vi "MergeOverrideViWithMethod.vi"(0 "ViRef":refnum<vi>, 1 "OverrideVIRef":refnum<vi>, 2 "GetControlNamesThatShouldBeIgnored":string[](array[string]), 5 "error in":errorcluster) -> (19 "error out":errorcluster)   [LabVIEW 2020, in "ClassWriterNative.lvclass"]
uses:
  <resource>/Framework/Providers/Open_GDS/ClassProviders/Provider_LvNativeClass/ClassWriterNative_class/ClassWriterNative.lvclass
  <vilib>/Utility/miscctls.llb/LVPositionTypeDef.ctl
  <resource>/Framework/Providers/Open_GDS/ClassProviders/Provider_LvNativeClass/ClassWriterNative_class/ClassWriterNative.lvclass/ClassWriterNative.ctl
  <userlib>/_OpenG.lib/error/error.llb/openg_error.lvlib
panel:
  out "These CP Termibnlas should not be connected to an controls":i32[](array[numeric])
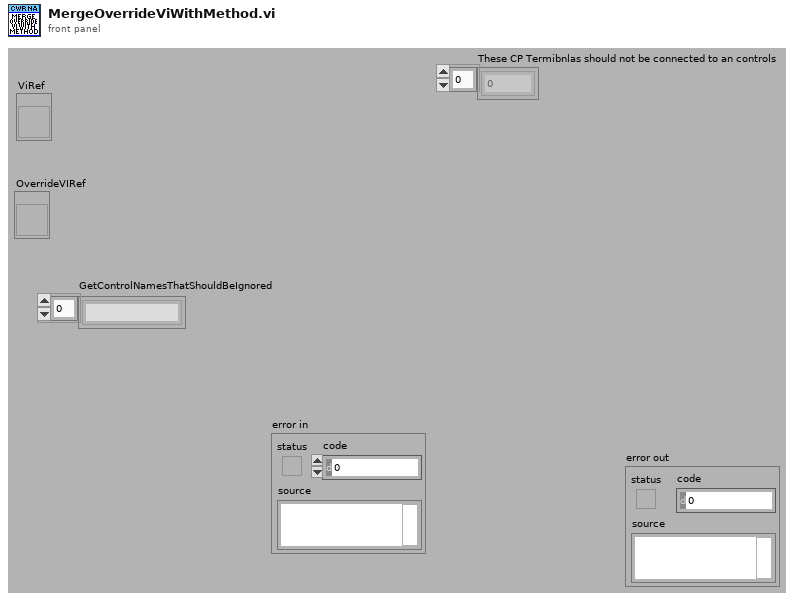
[diagram p1: front panel]
types:
  T1 = enum32{"invalid execution system", "user interface", "standard", "instrument i/o", "data acquisition", "other 1", "other 2", "same as caller"}
  T2 = enum32{"invalid priority", "background priority", "normal priority", "above normal priority", "high priority", "time critical priority", "subroutine"}
  T3 = enum16{"Share clones between instances", "Preallocate clone for each instance"}
  T4 = enum16{"Invalid Wire Rule", "Required", "Recommended", "Optional", "Dynamic Dispatch"}[]
  T5 = typedef "LVRectTypeDef.ctl" = cluster{"Left":i16, "Top":i16, "Right":i16, "Bottom":i16}
  T6 = typedef "LVPositionTypeDef.ctl" = cluster{"Left":i32, "Top":i32}
  T7 = enum16{"Invalid Wire Rule", "Required", "Recommended", "Optional", "Dynamic Dispatch"}
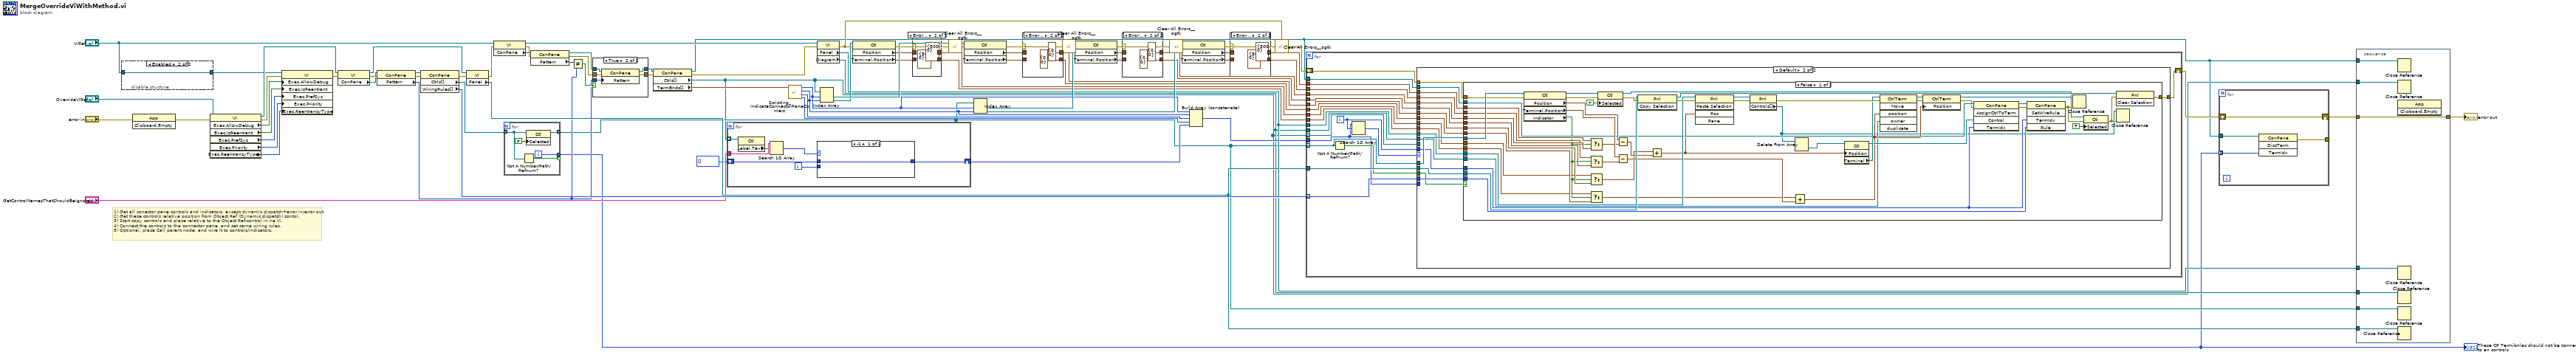
[diagram p0: block diagram]
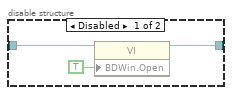
[diagram p6: hidden frame]
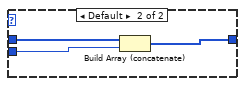
[diagram p8: hidden frame]
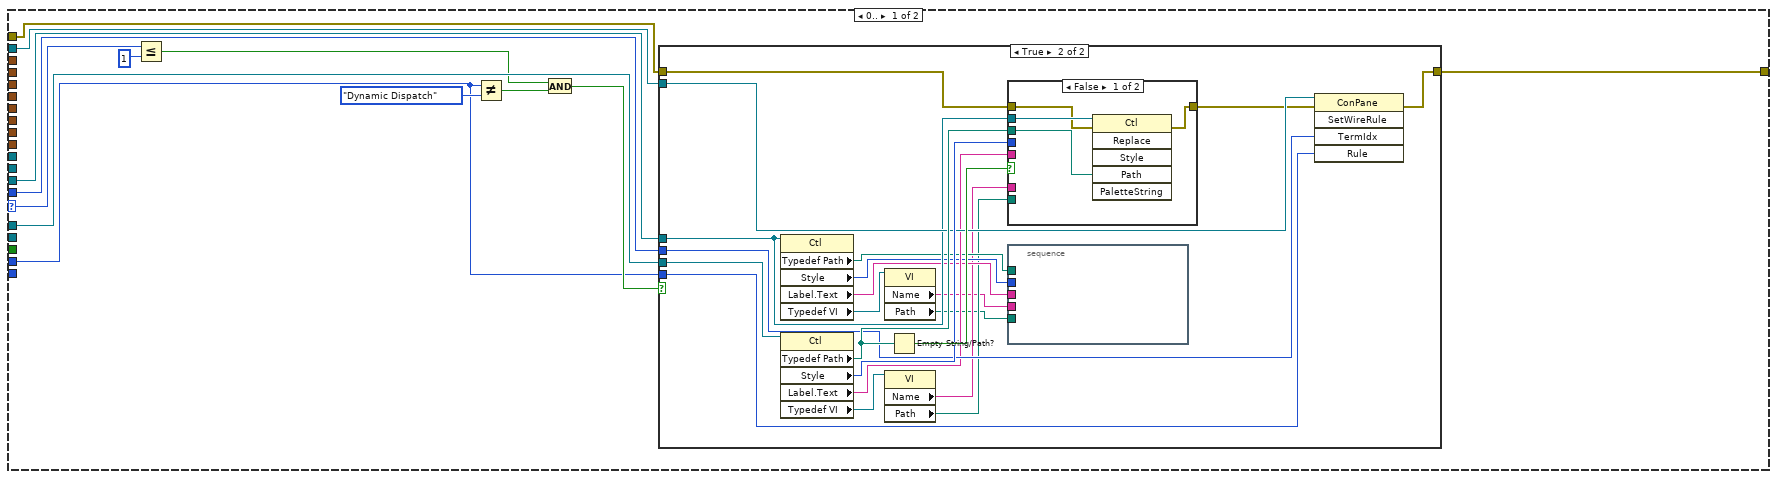
[diagram p9: hidden frame]
diagram:
  # "1) Get all conector pane controls and indicators, except dynamic dispatch+error in/error out\n2) Get these controls relative position from Object Ref (Dynamic dispatch) contol.\n3) Start copy controls and place relative to the Object Ref-control in ne VI.\n4) Connect the controls to the connector pane, and set same wiring rules.\n5) Optional. place Call parent node, and wire it to controls/indicators."
  n1 = disable-structure shown="Enabled" {
    disable-tunnel: "ViRef" -> [w84 w85]
    disable-tunnel: [w82 w85] -> w38
    frame Disabled {
      n2 = property class="VI"(reference=w84, "BDWin.Open"=TRUE ("Block Diagram Window:Open")) -> (reference out=w82:refnum<vi>)  [unwired: 1 in, 1 out]
    }
    frame Enabled {
    }
  }
  n3 = invoke class="App" method="Clipboard.Empty"(error in="error in") -> (error out=w34:errorcluster)  [unwired: 2 in, 2 out]
  n4 = property class="VI"(reference="OverrideVIRef", error in=w34) -> (reference out=w55:refnum<vi>, error out=w62:errorcluster, "Exec.AllowDebug"=w60:bool, "Exec.IsReentrant"=w59:bool, "Exec.PrefSys"=w58:T1, "Exec.Priority"=w57:T2, "Exec.ReentrancyType"=w56:T3)
  n5 = property class="VI"(reference=w38, error in=w62, "Exec.AllowDebug"=w60, "Exec.IsReentrant"=w59, "Exec.PrefSys"=w58, "Exec.Priority"=w57, "Exec.ReentrancyType"=w56) -> (error out=w61:errorcluster)  [unwired: 1 out]
  n6 = property class="VI"(reference=w55, error in=w61) -> (reference out=w71:refnum<vi>, error out=w54:errorcluster, "ConPane"=w52:refnum<vi>)
  n7 = property class="ConPane"(reference=w52, error in=w54) -> (reference out=w51:refnum<vi>, error out=w53:errorcluster, "Pattern"=w42:u32)
  n8 = property class="ConPane"(reference=w51, error in=w53) -> (error out=w72:errorcluster, "Ctrls[]"=w32:refnum<vi>[], "WiringRules[]"=w80:T4)  [unwired: 1 out]
  n9 = property class="VI"(reference=w71, error in=w72) -> (error out=w70:errorcluster, "Panel"=w73:refnum<vi>)  [unwired: 1 out]
  n10 = property class="VI"(reference="ViRef", error in=w70) -> (reference out=w81:refnum<vi>, error out=w47:errorcluster, "ConPane"=w48:refnum<vi>)
  n11 = for {
    tunnel: w32 -> [w88] mode=indexing
    tunnel: [w89] -> w31 mode=indexing
    tunnel: [w87] -> w2 mode=indexing if=w86
    i -> [w87]
    n12 = Not A Number/Path/Refnum?(number/path/refnum=w88) -> (NaN/Path/Refnum?=w86:bool)
    n13 = property class="Ctl"(reference=w88, "Selected"=FALSE) -> (reference out=w89:refnum<vi>)  [unwired: 1 in, 1 out]
  }
  "These CP Termibnlas should not be connected to an controls" <- w2
  n14 = property class="ConPane"(reference=w48, error in=w47) -> (reference out=w46:refnum<vi>, error out=w45:errorcluster, "Pattern"=w44:u32)
  n15 = Not Equal?(x=w44, y=w42) -> (x != y?=w43:bool)
  n16 = case shown="True" w43 {
    tunnel: [w92 w97] -> w50
    tunnel: [w91 w96] -> w49
    tunnel: w46 -> [w92 w95]
    tunnel: w45 -> [w91 w94]
    tunnel: w42 -> [_ w93]
    frame False {
    }
    frame True {
      n17 = property class="ConPane"(reference=w95, error in=w94, "Pattern"=w93) -> (reference out=w97:refnum<vi>, error out=w96:errorcluster)
    }
  }
  n18 = property class="ConPane"(reference=w50, error in=w49) -> (reference out=w1:refnum<vi>, error out=w37:errorcluster, "Ctrls[]"=w3:refnum<vi>[], "TermBnds[]"=w69:T5[])
  n19 = for {
    tunnel: w3 -> [w104] mode=indexing
    shift-right: [w102] -> w64
    shift-left: i32[] [] -> [w103]
    tunnel: "GetControlNamesThatShouldBeIgnored" -> [w100]
    i -> [w101]
    n20 = property class="Ctl"(reference=w104) -> ("Label.Text"=w99:string)  [unwired: 1 in, 2 out]
    n21 = Search 1D Array(1D array=w100, element=w99) -> (index of element=w98:i32)  [unwired: 1 in]
    n22 = case shown="-1" w98 {
      tunnel: w103 -> [w105 w108]
      tunnel: [w105 w107] -> w102
      tunnel: w101 -> [_ w106]
      frame -1 {
      }
      frame Default {
        n23 = Build Array (concatenate)(w108, w106) -> (w107:i32[])
      }
    }
  }
  n24 = call <resource>:"Scripting_IndicateConnectorPaneCorners.vi"("TermBnds[]"=w69) -> ("RightLower"=w67:i32, "LeftLower"=w68:i32, "RightTop"=w40:i32, "LeftTop"=w41:i32)  [unwired: 7 in]
  n25 = property class="VI"(reference=w81, error in=w37) -> (error out=w29:errorcluster, "Panel"=w74:refnum<vi>, "Diagram"=w36:refnum<vi>)  [unwired: 1 out]
  n26 = Index Array(array=w3, index #1=w41, index #2=w40) -> (element #1=w78:refnum<vi>, element #2=w77:refnum<vi>)
  n27 = property class="Ctl"(reference=w77, error in=w29) -> (error out=w25:errorcluster, "Position"=w24:T6, "Terminal.Position"=w23:T6)  [unwired: 1 out]
  n28 = case shown="Error .." w25 {
    tunnel: w24 -> [w110 _]
    tunnel: w23 -> [w109 _]
    tunnel: [w110 T6 {"Left"=500, "Top"=0} ("Position")] -> w22
    tunnel: [w109 T6 {"Left"=500, "Top"=0} ("Terminal.Position")] -> w21
    frame No Error {
    }
    frame Error {
    }
  }
  n29 = call <userlib>:"Clear All Errors__ogtk.vi"("Error In"=w25) -> ("Error Out"=w28:errorcluster)  [unwired: 3 in]
  n30 = property class="Ctl"(reference=w78, error in=w28) -> (error out=w20:errorcluster, "Position"=w19:T6, "Terminal.Position"=w17:T6)  [unwired: 1 out]
  n31 = Index Array(array=w31, index #1=w41, index #2=w40) -> (element #1=w79:refnum<vi>, element #2=w76:refnum<vi>)
  n32 = case shown="Error .." w20 {
    tunnel: w19 -> [w114 _]
    tunnel: w17 -> [w113 _]
    tunnel: [w114 T6 {"Left"=0, "Top"=0} ("Position")] -> w18
    tunnel: [w113 T6 {"Left"=0, "Top"=0} ("Terminal.Position")] -> w16
    frame No Error {
    }
    frame Error {
    }
  }
  n33 = call <userlib>:"Clear All Errors__ogtk.vi"("Error In"=w20) -> ("Error Out"=w27:errorcluster)  [unwired: 3 in]
  n34 = property class="Ctl"(reference=w79, error in=w27) -> (error out=w15:errorcluster, "Position"=w14:T6, "Terminal.Position"=w13:T6)  [unwired: 1 out]
  n35 = case shown="Error .." w15 {
    tunnel: w14 -> [w118 _]
    tunnel: w13 -> [w117 _]
    tunnel: [w118 T6 {"Left"=0, "Top"=0} ("Position")] -> w12
    tunnel: [w117 T6 {"Left"=0, "Top"=0} ("Terminal.Position")] -> w11
    frame No Error {
    }
    frame Error {
    }
  }
  n36 = call <userlib>:"Clear All Errors__ogtk.vi"("Error In"=w15) -> ("Error Out"=w26:errorcluster)  [unwired: 3 in]
  n37 = property class="Ctl"(reference=w76, error in=w26) -> (error out=w10:errorcluster, "Position"=w9:T6, "Terminal.Position"=w8:T6)  [unwired: 1 out]
  n38 = Build Array (concatenate)(w41, w40, w68, w67, w64) -> (w66:i32[])
  n39 = case shown="Error .." w10 {
    tunnel: w9 -> [w122 _]
    tunnel: w8 -> [w121 _]
    tunnel: [w122 T6 {"Left"=500, "Top"=0} ("Position")] -> w7
    tunnel: [w121 T6 {"Left"=500, "Top"=0} ("Terminal.Position")] -> w6
    frame No Error {
    }
    frame Error {
    }
  }
  n40 = call <userlib>:"Clear All Errors__ogtk.vi"("Upsteam Error (optional)"=w29, "Error In"=w10) -> ("Error Out"=w30:errorcluster)  [unwired: 2 in]
  n41 = for {
    tunnel: w31 -> [w145] mode=indexing
    tunnel: w12 -> [w137]
    tunnel: w11 -> [w136]
    tunnel: w73 -> [w144]
    tunnel: w74 -> [w143]
    tunnel: w18 -> [w134]
    tunnel: w16 -> [w133]
    tunnel: w1 -> [w142]
    tunnel: w80 -> [w129] mode=indexing
    shift-right: [w139] -> w5
    shift-left: w30 -> [w140]
    tunnel: w7 -> [w138]
    tunnel: w6 -> [w135]
    tunnel: w22 -> [w132]
    tunnel: w21 -> [w131]
    tunnel: w66 -> [w126]
    tunnel: w3 -> [w127] mode=indexing
    tunnel: w36 -> [w125]
    i -> [w128]
    n42 = Not A Number/Path/Refnum?(number/path/refnum=w145) -> (NaN/Path/Refnum?=w141:bool)
    n43 = Search 1D Array(1D array=w126, element=w128) -> (index of element=w130:i32)  [unwired: 1 in]
    n44 = case shown="Default" w130 {
      selector: w130 -> [w146 _]
      tunnel: w145 -> [w152 w203]
      tunnel: w144 -> [_ w202]
      tunnel: w143 -> [_ w201]
      tunnel: w142 -> [w151 w200]
      tunnel: w129 -> [w150 w199]
      tunnel: w141 -> [_ w198]
      tunnel: w140 -> [w155 w197]
      tunnel: [w154 w196] -> w139
      tunnel: w138 -> [_ w195]
      tunnel: w137 -> [_ w194]
      tunnel: w136 -> [_ w193]
      tunnel: w135 -> [_ w192]
      tunnel: w134 -> [_ w191]
      tunnel: w133 -> [_ w190]
      tunnel: w132 -> [_ w189]
      tunnel: w131 -> [_ w188]
      tunnel: w128 -> [w147 w187]
      tunnel: w127 -> [w153 _]
      tunnel: w126 -> [_ _]
      tunnel: w125 -> [_ w186]
      frame 0.. {
        n45 = Less Or Equal?(x=w146, y=1) -> (x <= y?=w148:bool)
        n46 = Not Equal?(x=w150, y=T7."Dynamic Dispatch") -> (x != y?=w157:bool)
        n47 = And(x=w148, y=w157) -> (x .and. y?=w156:bool)
        n48 = case shown="True" w156 {
          tunnel: w155 -> [w159 w180]
          tunnel: [w159 w174] -> w154
          tunnel: w153 -> [_ w169]
          tunnel: w152 -> [_ w171]
          tunnel: w151 -> [_ w176]
          tunnel: w150 -> [_ w173]
          tunnel: w147 -> [_ w172]
          frame False {
          }
          frame True {
            n49 = property class="Ctl"(reference=w169) -> ("Typedef Path"=w168:path, "Style"=w167:u32, "Label.Text"=w166:string, "Typedef VI"=w162:refnum<vi>)  [unwired: 1 in, 2 out]
            n50 = property class="Ctl"(reference=w171) -> ("Typedef Path"=w179:path, "Style"=w177:u32, "Label.Text"=w170:string, "Typedef VI"=w165:refnum<vi>)  [unwired: 1 in, 2 out]
            n51 = property class="VI"(reference=w162) -> ("Name"=w161:string, "Path"=w160:path)  [unwired: 1 in, 2 out]
            n52 = property class="VI"(reference=w165) -> ("Name"=w164:string, "Path"=w163:path)  [unwired: 1 in, 2 out]
            n53 = Empty String/Path?(string/path=w179) -> (empty?=w178:bool)
            n54 = case shown="False" w178 {
              tunnel: w169 -> [w184 _]
              tunnel: w180 -> [w183 w185]
              tunnel: w179 -> [w182 _]
              tunnel: [w181 w185] -> w175
              tunnel: w177 -> [_ _]
              tunnel: w170 -> [_ _]
              tunnel: w164 -> [_ _]
              tunnel: w163 -> [_ _]
              frame False {
                n55 = invoke class="Ctl" method="Replace"(reference=w184, error in=w183, "Path"=w182) -> (error out=w181:errorcluster)  [unwired: 3 in, 5 out]
              }
              frame True {
              }
            }
            n56 = stacked-sequence {
              tunnel: w168 -> [_]
              tunnel: w167 -> [_]
              tunnel: w166 -> [_]
              tunnel: w161 -> [_]
              tunnel: w160 -> [_]
              frame #0 {
              }
            }
            n57 = invoke class="ConPane" method="SetWireRule"(reference=w176, error in=w175, "TermIdx"=w172, "Rule"=w173) -> (error out=w174:errorcluster)  [unwired: 1 in, 4 out]
          }
        }
      }
      frame Default {
        n58 = case shown="False" w198 {
          tunnel: w203 -> [w252 _]
          tunnel: w202 -> [w248 _]
          tunnel: w201 -> [w247 _]
          tunnel: w200 -> [w243 _]
          tunnel: w199 -> [w241 _]
          tunnel: w187 -> [w208 _]
          tunnel: w197 -> [w240 w255]
          tunnel: [w220 w255] -> w196
          tunnel: w195 -> [w230 _]
          tunnel: w194 -> [w229 _]
          tunnel: w193 -> [w226 _]
          tunnel: w192 -> [w225 _]
          tunnel: w191 -> [w222 _]
          tunnel: w190 -> [w221 _]
          tunnel: w189 -> [w219 _]
          tunnel: w188 -> [w218 _]
          tunnel: w186 -> [w206 _]
          frame False {
            n59 = property class="Ctl"(reference=w252, error in=w240) -> (reference out=w251:refnum<vi>, error out=w239:errorcluster, "Position"=w254:T6, "Terminal.Position"=w253:T6, "Indicator"=w214:bool)
            n60 = Select(t=w230, s=w214, f=w229) -> (s? t:f=w228:T6)
            n61 = Select(t=w225, s=w214, f=w226) -> (s? t:f=w227:T6)
            n62 = Select(t=w219, s=w214, f=w222) -> (s? t:f=w223:T6)
            n63 = Select(t=w218, s=w214, f=w221) -> (s? t:f=w224:T6)
            n64 = property class="Ctl"(reference=w251, error in=w239, "Selected"=TRUE) -> (reference out=w216:refnum<vi>, error out=w249:errorcluster)
            n65 = Subtract(x=w254, y=w228) -> (x-y=w245:T6)
            n66 = Subtract(x=w253, y=w227) -> (x-y=w244:T6)
            n67 = invoke class="Pnl" method="Copy Selection"(reference=w248, error in=w249) -> (reference out=w234:refnum<vi>, error out=w246:errorcluster)  [unwired: 1 in, 1 out]
            n68 = Add(x=w223, y=w245) -> (x+y=w231:T6)
            n69 = invoke class="Pnl" method="Paste Selection"(reference=w247, error in=w246, "Pos"=w231) -> (reference out=w207:refnum<vi>, error out=w232:errorcluster)  [unwired: 2 in, 3 out]
            n70 = property class="Pnl"(reference=w207, error in=w232) -> (error out=w238:errorcluster, "Controls[]"=w205:refnum<vi>[])  [unwired: 1 out]
            n71 = Add(x=w224, y=w244) -> (x+y=w212:T6)
            n72 = Delete From Array(array=w205) -> (deleted portion=w233:refnum<vi>)  [unwired: 2 in, 1 out]
            n73 = property class="Ctl"(reference=w233, "Position"=w231) -> (reference out=w235:refnum<vi>, "Terminal"=w236:refnum<vi>)  [unwired: 1 in, 1 out]
            n74 = invoke class="CtrlTerm" method="Move"(reference=w236, error in=w238, "position"=w212, "owner"=w206) -> (reference out=w211:refnum<vi>, error out=w213:errorcluster)  [unwired: 2 in, 4 out]
            n75 = property class="CtrlTerm"(reference=w211, error in=w213, "Position"=w212) -> (reference out=w210:refnum<vi>, error out=w209:errorcluster)
            n76 = invoke class="ConPane" method="AssignCtrlToTerm"(reference=w243, error in=w209, "Control"=w235, "TermIdx"=w208) -> (reference out=w242:refnum<vi>, error out=w237:errorcluster)  [unwired: 1 in, 3 out]
            n77 = invoke class="ConPane" method="SetWireRule"(reference=w242, error in=w237, "TermIdx"=w208, "Rule"=w241) -> (error out=w215:errorcluster)  [unwired: 1 in, 4 out]
            n78 = Close Reference(reference=w210, error in (no error)=w215) -> ()  [unwired: 1 out]
            n79 = property class="Ctl"(reference=w216, error in=w215, "Selected"=FALSE) -> (error out=w204:errorcluster)  [unwired: 1 out]
            n80 = invoke class="Pnl" method="Clear Selection"(reference=w234, error in=w204) -> (error out=w220:errorcluster)  [unwired: 1 in, 2 out]
            n81 = Close Reference(reference=w205, error in (no error)=w204) -> ()  [unwired: 1 out]
          }
          frame True {
          }
        }
      }
    }
  }
  n82 = for {
    shift-right: [w259] -> w4
    shift-left: w5 -> [w259]
    tunnel: w2 -> [w258] mode=indexing
    tunnel: w1 -> [w257]
    tunnel: [w256] -> _
    n83 = invoke class="ConPane" method="DiscTerm"(reference=w257, "TermIdx"=w258) -> (error out=w256:errorcluster)  [unwired: 2 in, 3 out]
  }
  n84 = stacked-sequence {
    tunnel: w4 -> [w266]
    tunnel: [w266] -> w75
    tunnel: w31 -> [w261]
    tunnel: w3 -> [w262]
    tunnel: w1 -> [w265]
    tunnel: w74 -> [w264]
    tunnel: w73 -> [w263]
    tunnel: w36 -> [w260]
    frame #0 {
      n85 = Close Reference(reference=w265) -> ()  [unwired: 1 in, 1 out]
      n86 = Close Reference(reference=w262) -> ()  [unwired: 1 in, 1 out]
      n87 = Close Reference(reference=w264) -> ()  [unwired: 1 in, 1 out]
      n88 = Close Reference(reference=w260) -> ()  [unwired: 1 in, 1 out]
      n89 = Close Reference(reference=w261) -> ()  [unwired: 1 in, 1 out]
      n90 = Close Reference(reference=w263) -> ()  [unwired: 1 in, 1 out]
      n91 = invoke class="App" method="Clipboard.Empty"() -> ()  [unwired: 3 in, 3 out]
    }
  }
  "error out" <- w75
